vi "SendMsg.vi"(6 "Command response delay":dbl format="%#_6p", 7 "MsgType":T1=enum."DATA", 8 "error in":errorcluster, 10 "Payload":u16 format="%.0x", 11 "FPGA VI Reference In":refnum<k20>) -> (0 "error out":errorcluster, 2 "Data Received":u64[](array[numeric]) format="%.0x", 3 "FPGA VI Reference Out":refnum<k20>)   [LabVIEW 2019]
uses:
  TypeDefs/Type of message.ctl
  <vilib>/Utility/error.llb/Error Cluster From Error Code.vi
  <vilib>/rvi/errors/niLvFpgaAdjustHostInterfaceError.vi
  <vilib>/rvi/interface/nirviMethod/nirviMethod.xnode
  <vilib>/FPGAPlugInAG/Dynamic/niLvFpga_WriteFifo_Dynamic.vi
  <vilib>/rvi/errors/niLvFpgaMergeErrorWithErrorCode.vi
  <vilib>/FPGAPlugInAG/Dynamic/niLvFpga_ReadFifo_Dynamic.vi
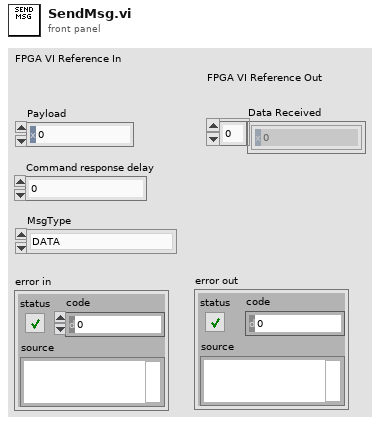
[diagram p1: front panel]
types:
  T1 = typedef "Type of message.ctl" = enum16{"CMD", "DATA"}
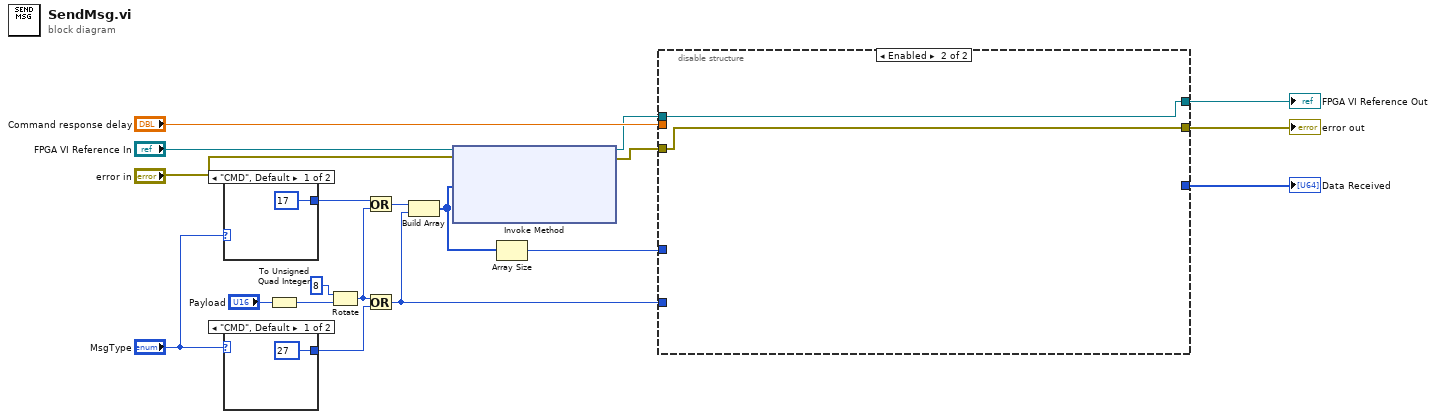
[diagram p0: block diagram]
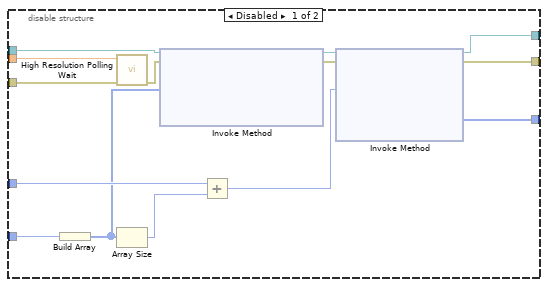
[diagram p2: hidden frame]
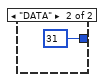
[diagram p3: hidden frame]
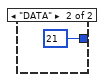
[diagram p4: hidden frame]
diagram:
  n1 = case shown="\"CMD\", Default" "MsgType" {
    tunnel: [u64 17 ("element") u64 21 ("element")] -> w9
    frame "CMD", Default {
    }
    frame "DATA" {
    }
  }
  n2 = case shown="\"CMD\", Default" "MsgType" {
    tunnel: [u64 27 ("element") u64 31 ("element")] -> w6
    frame "CMD", Default {
    }
    frame "DATA" {
    }
  }
  n3 = To Unsigned Quad Integer(1:"Payload") -> (0:w5:u64)
  n4 = Rotate(1:w5, 2:i16 8 ("y")) -> (0:w4:u64)
  n5 = Or(x=w9, y=w4) -> (x .or. y?=w8:u64)
  n6 = Or(x=w4, y=w6) -> (x .or. y?=w1:u64)
  n7 = Build Array(w8, w1) -> (w7:u64[])
  n8 = xnode "Invoke Method"("FPGA VI Reference In"="FPGA VI Reference In", "error in"="error in", "Data"=w7) -> ("FPGA VI Reference Out"=w16:refnum<k20>, "error out"=w18:errorcluster)  [unwired: 1 in, 1 out]
  n9 = Array Size(array=w7) -> (size(s)=w12:i32)
  n10 = disable-structure shown="Enabled" {
    disable-tunnel: w18 -> [w37 w39]
    disable-tunnel: "Command response delay" -> [w36 _]
    disable-tunnel: w16 -> [w35 w38]
    disable-tunnel: [w31 w38] -> w13
    disable-tunnel: w12 -> [w30 _]
    disable-tunnel: [w27 w39] -> w11
    disable-tunnel: [w26 _] -> w10
    disable-tunnel: w1 -> [w24 _]
    frame Disabled {
      n11 = Build Array(w24) -> (w25:u64[])
      n12 = call <vilib>:"High Resolution Polling Wait.vi"("error in (no error)"=w37, "seconds to wait"=w36) -> ("error out"=w34:errorcluster)  [unwired: 9 in]
      n13 = Array Size(array=w25) -> (size(s)=w29:i32)
      n14 = xnode "Invoke Method"("FPGA VI Reference In"=w35, "error in"=w34, "Data"=w25) -> ("FPGA VI Reference Out"=w32:refnum<k20>, "error out"=w33:errorcluster)  [unwired: 1 in, 1 out]
      n15 = Add(x=w30, y=w29) -> (x+y=w28:i32)
      n16 = xnode "Invoke Method"("FPGA VI Reference In"=w32, "error in"=w33, "Number of Elements"=w28) -> ("FPGA VI Reference Out"=w31:refnum<k20>, "error out"=w27:errorcluster, "Data"=w26:u64[])  [unwired: 1 in, 1 out]
    }
    frame Enabled {
    }
  }
  "FPGA VI Reference Out" <- w13
  "error out" <- w11
  "Data Received" <- w10
